vi "crossProduct.vi"(3 "B":dbl[](array[numeric]), 5 "A":dbl[](array[numeric])) -> (1 "A x B":dbl[](array[numeric]))   [LabVIEW 2013]
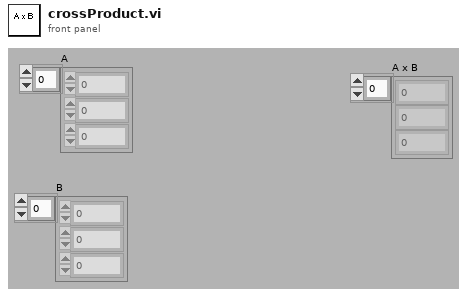
[diagram p1: front panel]
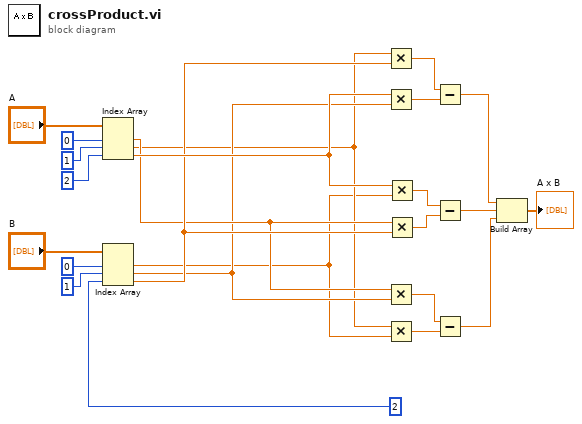
[diagram p0: block diagram]
diagram:
  n1 = Index Array(array="A", index #1=0 ("index"), index #2=1 ("index"), index #3=2 ("index")) -> (element #1=w10:dbl, element #2=w8:dbl, element #3=w14:dbl)
  n2 = Index Array(array="B", index #1=0 ("index"), index #2=1 ("index"), index #3=2 ("index")) -> (element #1=w7:dbl, element #2=w9:dbl, element #3=w13:dbl)
  n3 = Multiply(x=w8, y=w13) -> (x*y=w16:dbl)
  n4 = Multiply(x=w14, y=w9) -> (x*y=w15:dbl)
  n5 = Multiply(x=w10, y=w9) -> (x*y=w6:dbl)
  n6 = Multiply(x=w8, y=w7) -> (x*y=w5:dbl)
  n7 = Multiply(x=w14, y=w7) -> (x*y=w12:dbl)
  n8 = Multiply(x=w10, y=w13) -> (x*y=w11:dbl)
  n9 = Subtract(x=w16, y=w15) -> (x-y=w4:dbl)
  n10 = Subtract(x=w12, y=w11) -> (x-y=w3:dbl)
  n11 = Subtract(x=w6, y=w5) -> (x-y=w2:dbl)
  n12 = Build Array(w4, w3, w2) -> (→"A x B":dbl[])
